vi "Setup Actuator.vi"(8 "error in (no error)":errorcluster, 10 "Model in":refnum<class "Model.lvclass">, 11 "Boot Loader in":refnum<class "Boot Loader.lvclass">) -> (0 "error out":errorcluster, 2 "Model out":refnum<class "Model.lvclass">, 3 "Boot Loader out":refnum<class "Boot Loader.lvclass">)   [LabVIEW 2015, in "Boot Loader.lvclass"]
uses:
  Boot Loader.lvclass
  Model/Model.lvclass
  Actuator/Actuator Factory/Actuator Factory.lvclass
  Model/Model.lvclass/Model.ctl
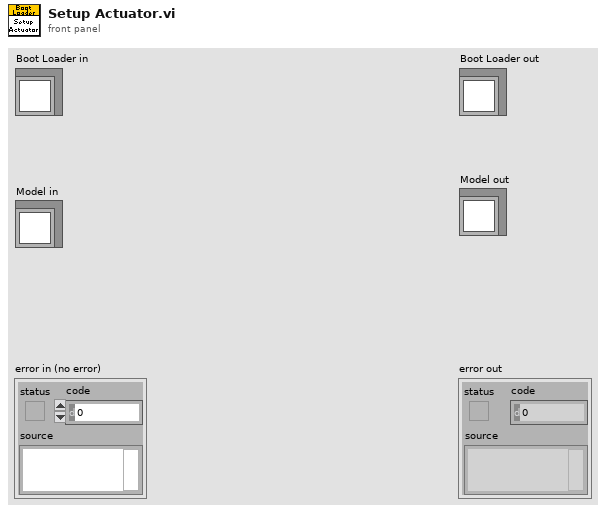
[diagram p1: front panel]
types:
  T1 = typedef "FAMT Typedefs.lvlib/Hardware Settings.ctl" = cluster{"Actuator Types":T2, "Cylinder Types":T3}
  T2 = typedef "FAMT Typedefs.lvlib/Actuator Types.ctl" = enum16{"Single", "Dual"}
  T3 = typedef "FAMT Typedefs.lvlib/Cylinder Types.ctl" = enum16{"PSV Open", "PSV Closed", "TV Open", "TV Closed", "Closed"}
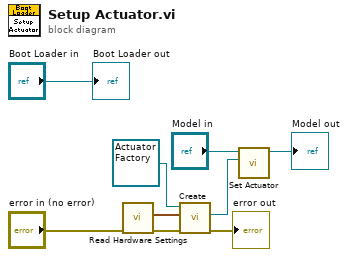
[diagram p0: block diagram]
diagram:
  n1 = call "Read Hardware Settings.vi"("error in (no error)"="error in (no error)") -> ("error out"=w3:errorcluster, "Hardware Settings"=w5:T1)  [unwired: 8 in, 1 out]
  n2 = call-dynamic "Create.vi"("error in (no error)"=w3, "Hardware Settings"=w5, "Actuator Factory in"=refnum<class "Actuator Factory.lvclass"> refnum ("ActuatorFactory.lvclass")) -> ("error out"=→"error out":errorcluster, "Actuator"=w1:refnum<class "Actuator.lvclass">)  [unwired: 6 in, 1 out]
  n3 = call "Set Actuator.vi"("Actuator.lvclass"=w1, "Model in"="Model in") -> ("Model out"=→"Model out":refnum<class "Model.lvclass">)  [unwired: 9 in]
  "Boot Loader out" <- "Boot Loader in"
